vi "Calibration.vi"() -> ()   [LabVIEW 2020]
panel:
  in  "saving path Template Calibrazione":path=path "C:/Users/Dell/Documents/Sistemi di visione/ProgrammiCompleti/Image/calib-info.png"
  out "error out":errorcluster
  in  "error in (no error)":errorcluster
  in  "Image Path":path=path "C:/Users/Dell/Documents/Sistemi di visione/ProgrammiCompleti/Image/CalibGrid_10mm.png"
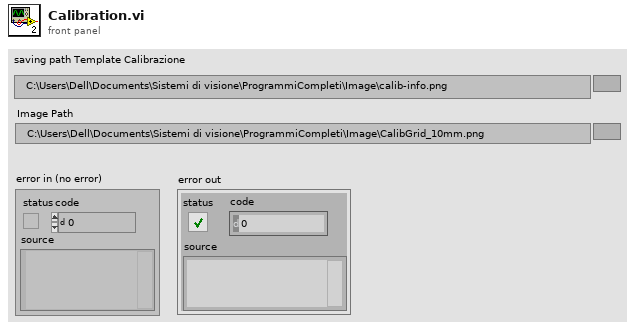
[diagram p1: front panel]
types:
  T1 = typedef "IMAQ Image.ctl" = refnum<image>
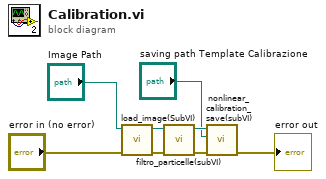
[diagram p0: block diagram]
diagram:
  n1 = call "load_image(SubVI).vi"("error in (no error)"="error in (no error)", "Image Path"="Image Path") -> ("error out"=w4:errorcluster, "Image GRAY"=w5:T1)  [unwired: 8 in]
  n2 = call "filtro_particelle(subVI).vi"("error in (no error)"=w4, "Image Src"=w5) -> ("error out"=w3:errorcluster, "Image"=w2:T1)  [unwired: 8 in]
  n3 = call "nonlinear_calibration_save(subVI).vi"("error in (no error)"=w3, "saving path Template Calibrazione"="saving path Template Calibrazione", "Image Src"=w2) -> ("error out"=→"error out":errorcluster)  [unwired: 6 in, 2 out]
